vi "Old_S2C_VAR_Initialize.vi"(8 "Error In":errorcluster, 11 "CtrlRef":refnum<vi>) -> (0 "Error Out":errorcluster)   [LabVIEW 2015]
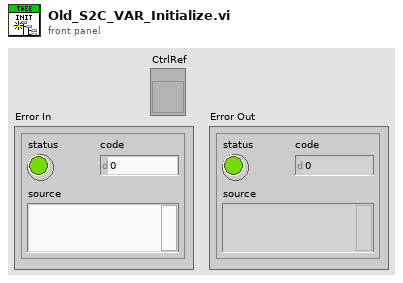
[diagram p1: front panel]
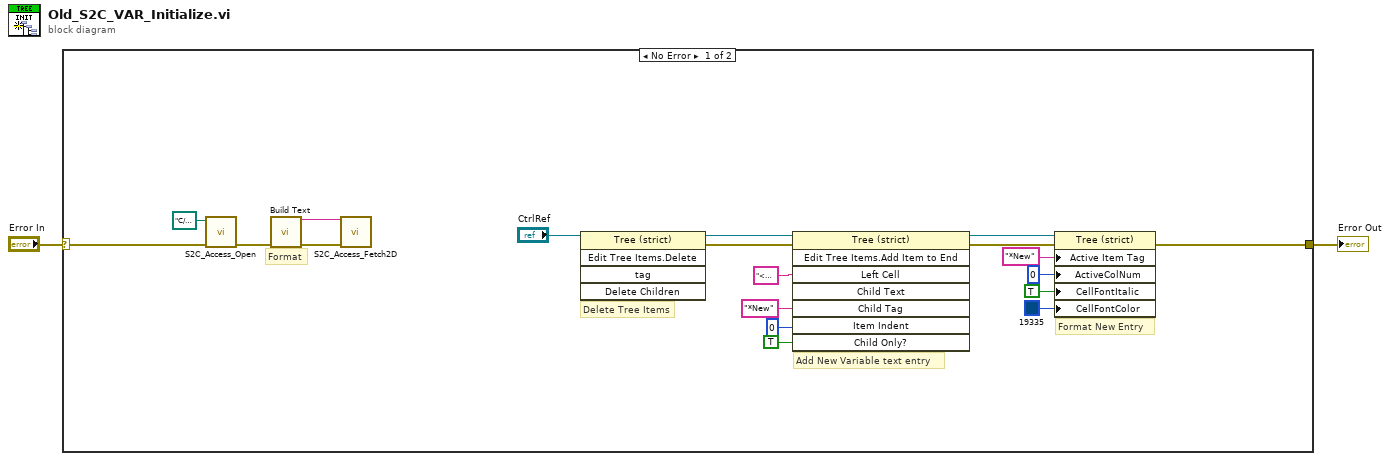
[diagram p0: block diagram]
diagram:
  n1 = case shown="No Error" "Error In" {
    selector: "Error In" -> [w7 w22]
    tunnel: [w10 w22] -> w1
    frame No Error {
      # "Format"
      # "Format New Entry"
      # "Add New Variable text entry"
      # "Delete Tree Items"
      n2 = call "S2C_Access_Open.vi"("Error In"=w7, "DSN_Path"=path "C:/Personal/Labview/S2C/AccessDB.dsn") -> ("Error Out"=w5:errorcluster)  [unwired: 8 in, 1 out]
      n3 = call "Build Text"("error in (no error)"=w5) -> ("Result"=w3:string, "error out"=w4:errorcluster)  [unwired: 13 in]
      n4 = call "S2C_Access_Fetch2D.vi"("Error In"=w4, "Query"=w3) -> ()  [unwired: 8 in, 2 out]
      n5 = invoke on="Invoke Node" class="Tree (strict)" method="Edit Tree Items.Delete"(reference="CtrlRef") -> (reference out=w9:refnum<vi>, error out=w17:errorcluster)  [unwired: 4 in, 3 out]
      n6 = invoke on="Invoke Node" class="Tree (strict)" method="Edit Tree Items.Add Item to End"(reference=w9, error in=w17, "Left Cell"="<Right-click for new variable>", "Child Tag"="*New", "Item Indent"=0 ("New Item Indentation"), "Child Only?"=TRUE) -> (reference out=w8:refnum<vi>, error out=w16:errorcluster)  [unwired: 2 in, 6 out]
      n7 = property on="Property Node" class="Tree (strict)"(reference=w8, error in=w16, "Active Item Tag"="*New", "ActiveColNum"=0 ("Active Cell:Active Column Number"), "CellFontItalic"=TRUE ("Active Cell:Cell Font:Italic"), "CellFontColor"=u32 19335) -> (error out=w10:errorcluster)  [unwired: 1 out]
    }
    frame Error {
    }
  }
  "Error Out" <- w1
